vi "AddSGL.vi"(10 "Y":u32=1106509824, 11 "X":u32=1106509824) -> (3 "Output":u32)   [LabVIEW 2016, in "FPGAMockHPILC.lvlib"]
uses:
  FPGAMockHPILC.lvlib
  <vilib>/rvi/Emulation/niFpgaGetClockAttributes.vi
  <vilib>/rvi/Emulation/niFpgaSctlEmulationGetInTimedLoop.vi
  <vilib>/rvi/Emulation/niFpgaEmulationReportErrorSimple.vi
  <vilib>/rvi/Emulation/niFpgaCriticalErrorInLSC.vi
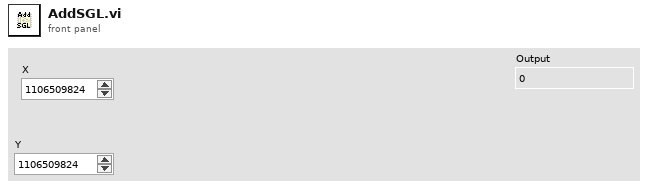
[diagram p1: front panel]
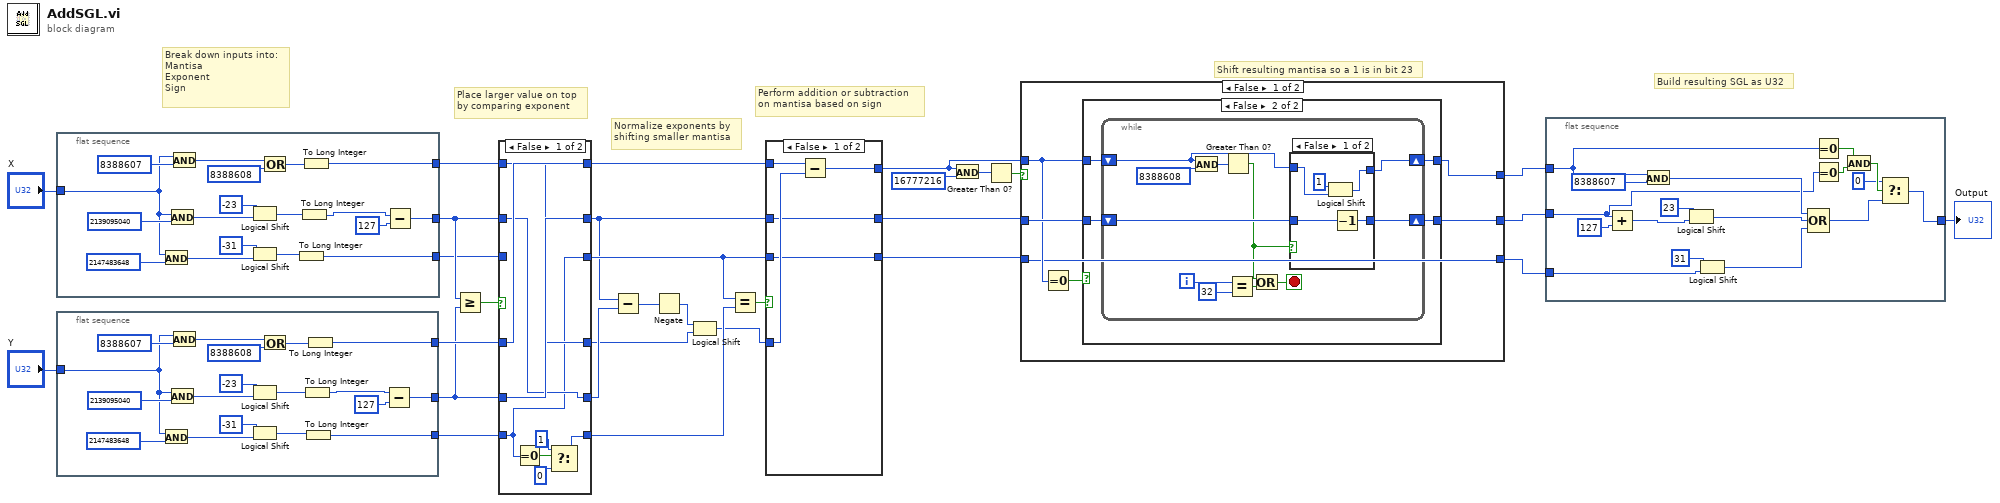
[diagram p0: block diagram]
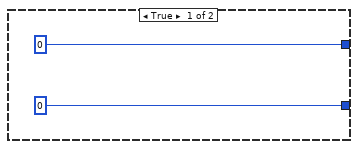
[diagram p2: hidden frame]
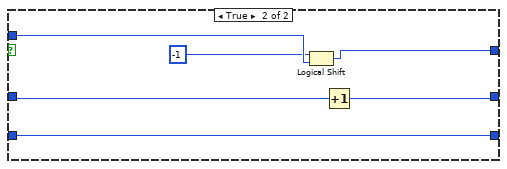
[diagram p4: hidden frame]
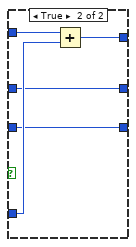
[diagram p6: hidden frame]
diagram:
  # "Build resulting SGL as U32"
  # "Shift resulting mantisa so a 1 is in bit 23"
  # "Perform addition or subtraction\non mantisa based on sign"
  # "Normalize exponents by\nshifting smaller mantisa"
  # "Place larger value on top\nby comparing exponent"
  # "Break down inputs into:\nMantisa\nExponent\nSign"
  n1 = flat-sequence {
    tunnel: "X" -> [w37]
    tunnel: [w36] -> w27
    tunnel: [w33] -> w28
    tunnel: [w30] -> w26
    frame #0 {
      n2 = And(x=w37, y=u32 2147483648) -> (x .and. y?=w39:u32)
      n3 = And(x=w37, y=u32 2139095040) -> (x .and. y?=w47:u32)
      n4 = And(x=w37, y=u32 8388607) -> (x .and. y?=w45:u32)
      n5 = Logical Shift(y=i16 -23, x=w47) -> (x << y=w35:u32)
      n6 = Logical Shift(y=i16 -31, x=w39) -> (x << y=w31:u32)
      n7 = Or(x=w45, y=u32 8388608) -> (x .or. y?=w34:u32)
      n8 = To Long Integer(number=w31) -> (32bit integer=w30:i32)
      n9 = To Long Integer(number=w35) -> (32bit integer=w32:i32)
      n10 = To Long Integer(number=w34) -> (32bit integer=w33:i32)
      n11 = Subtract(x=w32, y=127) -> (x-y=w36:i32)
    }
  }
  n12 = flat-sequence {
    tunnel: "Y" -> [w55]
    tunnel: [w54] -> w24
    tunnel: [w49] -> w23
    tunnel: [w48] -> w25
    frame #0 {
      n13 = And(x=w55, y=u32 2147483648) -> (x .and. y?=w57:u32)
      n14 = And(x=w55, y=u32 2139095040) -> (x .and. y?=w65:u32)
      n15 = And(x=w55, y=u32 8388607) -> (x .and. y?=w63:u32)
      n16 = Logical Shift(y=i16 -23, x=w65) -> (x << y=w51:u32)
      n17 = Logical Shift(y=i16 -31, x=w57) -> (x << y=w52:u32)
      n18 = Or(x=w63, y=u32 8388608) -> (x .or. y?=w53:u32)
      n19 = To Long Integer(number=w51) -> (32bit integer=w50:i32)
      n20 = To Long Integer(number=w52) -> (32bit integer=w49:i32)
      n21 = To Long Integer(number=w53) -> (32bit integer=w48:i32)
      n22 = Subtract(x=w50, y=127) -> (x-y=w54:i32)
    }
  }
  n23 = Greater Or Equal?(x=w27, y=w24) -> (x >= y?=w29:bool)
  n24 = case shown="False" w29 {
    tunnel: w28 -> [w72 w80]
    tunnel: w27 -> [w71 w79]
    tunnel: w26 -> [_ w78]
    tunnel: w25 -> [w74 w77]
    tunnel: w24 -> [w73 w76]
    tunnel: w23 -> [w70 w75]
    tunnel: [w74 w80] -> w20
    tunnel: [w73 w79] -> w16
    tunnel: [w70 w78] -> w19
    tunnel: [w72 w77] -> w14
    tunnel: [w71 w76] -> w15
    tunnel: [w66 w75] -> w22
    frame False {
      n25 = Equal To 0?(x=w70) -> (x = 0?=w69:bool)
      n26 = Select(t=1 ("y"), s=w69, f=0) -> (s? t:f=w66:i32)
    }
    frame True {
    }
  }
  n27 = Subtract(x=w16, y=w15) -> (x-y=w13:i32)
  n28 = Negate(x=w13) -> (-x=w12:i32)
  n29 = Logical Shift(y=w12, x=w14) -> (x << y=w11:i32)
  n30 = Equal?(x=w19, y=w22) -> (x = y?=w21:bool)
  n31 = case shown="False" w21 {
    tunnel: w20 -> [w84 w89]
    tunnel: w11 -> [w85 w90]
    tunnel: [w82 w88] -> w5
    tunnel: w19 -> [w82 w88]
    tunnel: [w83 w87] -> w2
    tunnel: [w81 w86] -> w4
    tunnel: w16 -> [w81 w86]
    frame False {
      n32 = Subtract(x=w84, y=w85) -> (x-y=w83:i32)
    }
    frame True {
      n33 = Add(x=w89, y=w90) -> (x+y=w87:i32)
    }
  }
  n34 = And(x=w2, y=16777216) -> (x .and. y?=w17:i32)
  n35 = Greater Than 0?(x=w17) -> (x > 0?=w3:bool)
  n36 = case shown="False" w3 {
    tunnel: w4 -> [w96 w122]
    tunnel: w2 -> [w93 w125]
    tunnel: [w95 w121] -> w8
    tunnel: w5 -> [w92 w126]
    tunnel: [w92 w126] -> w7
    tunnel: [w91 w123] -> w6
    frame False {
      n37 = Equal To 0?(x=w93) -> (x = 0?=w94:bool)
      n38 = case shown="False" w94 {
        tunnel: w93 -> [_ w102]
        tunnel: w96 -> [_ w101]
        tunnel: [0 w100] -> w95
        tunnel: [0 w99] -> w91
        frame True {
        }
        frame False {
          n39 = while {
            shift-right: [w103] -> w99
            shift-left: w102 -> [w104]
            shift-right: [w110] -> w100
            shift-left: w101 -> [w111]
            i -> [w109]
            stop <- w106 stop-if-true
            n40 = And(x=w104, y=8388608) -> (x .and. y?=w112:i32)
            n41 = Greater Than 0?(x=w112) -> (x > 0?=w105:bool)
            n42 = Equal?(x=w109, y=32) -> (x = y?=w107:bool)
            n43 = Or(x=w105, y=w107) -> (x .or. y?=w106:bool)
            n44 = case shown="False" w105 {
              tunnel: w104 -> [w116 w120]
              tunnel: w111 -> [w118 w119]
              tunnel: [w114 w120] -> w103
              tunnel: [w117 w119] -> w110
              frame False {
                n45 = Logical Shift(y=i16 1, x=w116) -> (x << y=w114:i32)
                n46 = Decrement(x=w118) -> (x-1=w117:i32)
              }
              frame True {
              }
            }
          }
        }
      }
    }
    frame True {
      n47 = Logical Shift(y=i16 -1, x=w125) -> (x << y=w123:i32)
      n48 = Increment(x=w122) -> (x+1=w121:i32)
    }
  }
  n49 = flat-sequence {
    tunnel: w8 -> [w128]
    tunnel: w7 -> [w139]
    tunnel: w6 -> [w127]
    tunnel: [w133] -> w1
    frame #0 {
      n50 = Add(x=w128, y=127) -> (x+y=w141:i32)
      n51 = And(x=w127, y=u32 8388607) -> (x .and. y?=w135:u32)
      n52 = Logical Shift(y=i16 23, x=w141) -> (x << y=w136:i32)
      n53 = Logical Shift(y=i16 31, x=w139) -> (x << y=w137:i32)
      n54 = Compound Arithmetic op=OR(w135, w136, w137) -> (w134:u32)
      n55 = Equal To 0?(x=w127) -> (x = 0?=w132:bool)
      n56 = Equal To 0?(x=w128) -> (x = 0?=w131:bool)
      n57 = And(x=w132, y=w131) -> (x .and. y?=w130:bool)
      n58 = Select(t=u32 0, s=w130, f=w134) -> (s? t:f=w133:u32)
    }
  }
  "Output" <- w1
